vi "filtro_particelle(subVI).vi"(5 "Look For (Dark Objects)":u32(ring)=1 items=["Bright Objects", "Dark Objects"], 7 "Window Size (32x32)":cluster{"SizeX":i32, "SizeY":i32}={"SizeX"=150, "SizeY"=150} {"SizeY" min=3 step=1; "SizeX" min=3 step=1}, 8 "error in (no error)":errorcluster, 10 "Selection Values":T3(array[cluster])=[{"Measurement Parameter"=35, "Range Lower Value"=0.0, "Range Upper Value"=15000.0, "Range"=FALSE, "Measurement Type"=FALSE}] {"Measurement Parameter" items=["Center of Mass X", "Center of Mass Y", "First Pixel X", "First Pixel Y", "Bounding Rect Left", "Bounding Rect Top", "Bounding Rect Right", "Bounding Rect Bottom", "Max Feret Diameter Start X", "Max Feret Diameter Start Y", "Max Feret Diameter End X", "Max Feret Diameter End Y", "Max Horiz. Segment Length Left", "Max Horiz. Segment Length Right", "Max Horiz. Segment Length Row", "-", "Bounding Rect Width", "Bounding Rect Height", "Bounding Rect Diagonal", "Perimeter", "Convex Hull Perimeter", "Holes' Perimeter", "Max Feret Diameter", "Equivalent Ellipse Major Axis", "Equivalent Ellipse Minor Axis", "Equivalent Ellipse Minor Axis (Feret)", "Equivalent Rect Long Side", "Equivalent Rect Short Side", "Equivalent Rect Diagonal", "Equivalent Rect Short Side (Feret)", "Average Horiz. Segment Length", "Average Vert. Segment Length", "Hydraulic Radius", "Waddel Disk Diameter", "-", "Area", "Holes' Area", "Particle & Holes' Area", "Convex Hull Area", "Image Area", "-", "Number of Holes", "Number of Horiz. Segments", "Number of Vert. Segments", "-", "Orientation", "Max Feret Diameter Orientation", "-", "% Area/Image Area", "% Area/(Particle & Holes' Area)", "Ratio of Equivalent Ellipse Axes", "Ratio of Equivalent Rect Sides", "-", "Elongation Factor", "Compactness Factor", "Heywood Circularity Factor", "Type Factor", "-", "Sum X", "Sum Y", "Sum XX", "Sum XY", "Sum YY", "Sum XXX", "Sum XXY", "Sum XYY", "Sum YYY", "-", "Moment of Inertia XX", "Moment of Inertia XY", "Moment of Inertia YY", "Moment of Inertia XXX", "Moment of Inertia XXY", "Moment of Inertia XYY", "Moment of Inertia YYY", "Norm. Moment of Inertia XX", "Norm. Moment of Inertia XY", "Norm. Moment of Inertia YY", "Norm. Moment of Inertia XXX", "Norm. Moment of Inertia XXY", "Norm. Moment of Inertia XYY", "Norm. Moment of Inertia YYY", "Hu Moment 1", "Hu Moment 2", "Hu Moment 3", "Hu Moment 4", "Hu Moment 5", "Hu Moment 6", "Hu Moment 7"]; "Range Lower Value" format="%.2f"; "Range Upper Value" format="%.2f"}, 11 "Image Src":T1=refnum) -> (0 "error out":errorcluster, 3 "Image 2":T1(plugin-control))   [LabVIEW 2020]
uses:
  <vilib>/vision/Image Controls.llb/IMAQ Image.ctl
  <vilib>/vision/NI_Vision_Development_Module.lvlib
panel:
  in  "Replace Value (1)":sgl=255.0 format="%.2f"
  in  "stop":bool
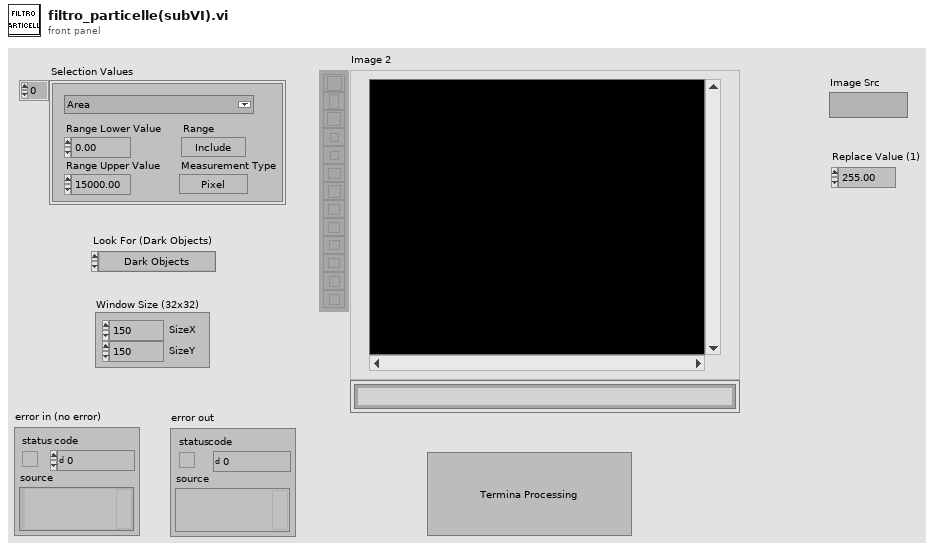
[diagram p1: front panel]
types:
  T1 = typedef "IMAQ Image.ctl" = refnum<image>
  T2 = typedef "Particle Parameters" = i32
  T3 = cluster{"Measurement Parameter":T2, "Range Lower Value":dbl, "Range Upper Value":dbl, "Range":bool, "Measurement Type":bool}[]
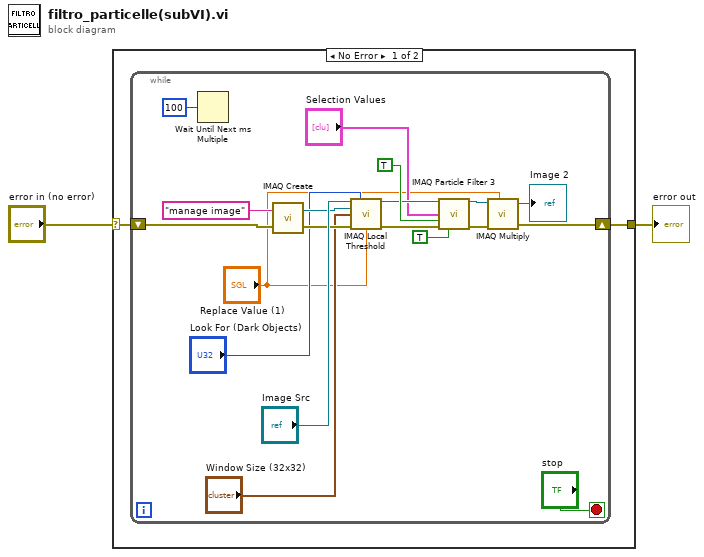
[diagram p0: block diagram]
diagram:
  n1 = case shown="No Error" "error in (no error)" {
    selector: "error in (no error)" -> [w3 w24]
    tunnel: [w4 w24] -> w2
    frame No Error {
      n2 = while {
        shift-right: [w7] -> w4
        shift-left: w3 -> [w17]
        stop <- "stop" stop-if-true
        n3 = Wait Until Next ms Multiple(millisecond multiple=u32 100) -> ()  [unwired: 1 out]
        n4 = call "IMAQ Create"("Image Name"="manage image", "error in (no error)"=w17) -> ("New Image"=w14:T1, "error out"=w16:errorcluster)  [unwired: 3 in]
        n5 = call "IMAQ Local Threshold"("Image Src"="Image Src", "Look For (Bright Objects)"="Look For (Dark Objects)", "Image Dst"=w14, "Window Size (32x32)"="Window Size (32x32)", "error in (no error)"=w16, "Replace Value (1)"="Replace Value (1)") -> ("Image Dst Out"=w20:T1, "error out"=w21:errorcluster)  [unwired: 8 in]
        n6 = call "IMAQ Particle Filter 3"("Image Src"=w20, "Selection Values"="Selection Values", "Keep/Remove Particles (F)"=TRUE, "error in (no error)"=w21, "Reject Border? (F)"=TRUE) -> ("Image Dst Out"=w9:T1, "error out"=w8:errorcluster)  [unwired: 8 in, 1 out]
        n7 = call "IMAQ Multiply"("Image Src A"=w9, "Constant"="Replace Value (1)", "error in (no error)"=w8) -> ("Image Dst Out"=→"Image 2":T1, "error out"=w7:errorcluster)  [unwired: 4 in]
      }
    }
    frame Error {
    }
  }
  "error out" <- w2
